vi "Climb Prep.vi"(10 "Start":bool, 11 "Enum":enum16{"Start", "Run", "End"}(ring)) -> (3 "Climb":bool)   [LabVIEW 2012]
uses:
  <vilib>/Rock Robotics/WPI/Solenoid/WPI_SolenoidValue.ctl
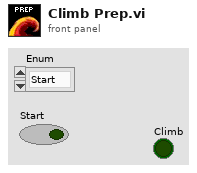
[diagram p1: front panel]
types:
  T1 = typedef "WPI_SolenoidValue.ctl" = enum16{"Off", "On", "Forward", "Reverse"}
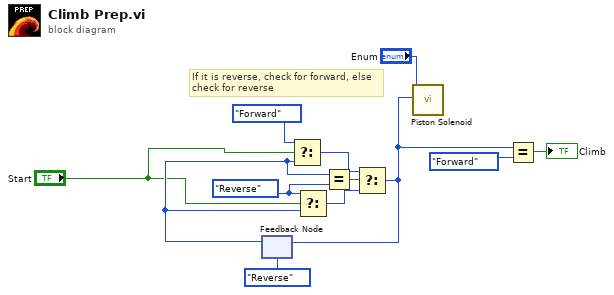
[diagram p0: block diagram]
diagram:
  w2 = WPI_SolenoidValue."Reverse" ("Value")
  # "If it is reverse, check for forward, else\ncheck for reverse"
  n1 = feedback #1(WPI_SolenoidValue."Reverse" ("Value")) -> (w3:T1)
  n2 = Select(t=WPI_SolenoidValue."Forward" ("Value"), s="Start", f=w3) -> (s? t:f=w9:T1)
  n3 = Select(t=w2, s="Start", f=w3) -> (s? t:f=w8:T1)
  n4 = Equal?(x=w3, y=w2) -> (x = y?=w10:bool)
  n5 = Select(t=w9, s=w10, f=w8) -> (s? t:f=w4:T1)
  n6 = feedback-in #1(w4) -> ()
  n7 = call "Piston Solenoid.vi"("Value"=w4, "Enum"="Enum") -> ()  [unwired: 10 in]
  n8 = Equal?(x=w4, y=WPI_SolenoidValue."Forward") -> (x = y?=→"Climb":bool)
